vi "Control states_X-Y.vi"(7 "Command":T1(ring), 8 "error in (no error)":errorcluster, 10 "Reference in":refnum<vi>[](array[refnum])) -> (0 "error out":errorcluster)   [LabVIEW 2018]
doc: "This VI is used to enable & disable the controls"
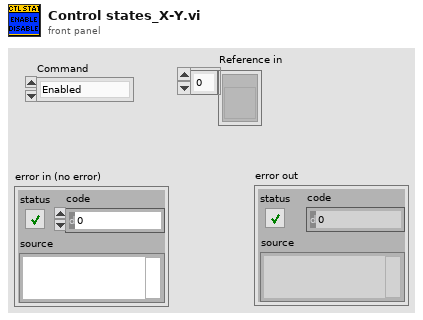
[diagram p1: front panel]
types:
  T1 = enum8{"Enabled", "Disabled", "Disabled and Grayed Out"}
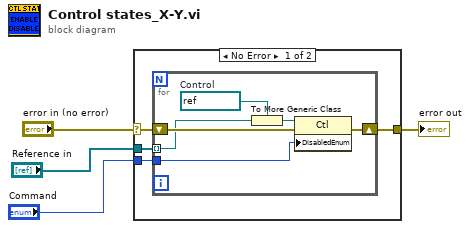
[diagram p0: block diagram]
diagram:
  n1 = case shown="No Error" "error in (no error)" {
    selector: "error in (no error)" -> [w8 w15]
    tunnel: [w7 w15] -> w3
    tunnel: "Reference in" -> [w6 _]
    tunnel: "Command" -> [w5 _]
    frame No Error {
      n2 = for {
        shift-right: [w13] -> w7
        shift-left: w8 -> [w14]
        tunnel: w6 -> [w11] mode=indexing
        tunnel: w5 -> [w9]
        w12 = refnum<vi> refnum  # Control
        n3 = To More Generic Class(target class=w12, reference=w11) -> (generic class reference=w10:refnum<vi>)
        n4 = property class="Ctl"(reference=w10, error in=w14, "DisabledEnum"=w9) -> (error out=w13:errorcluster)  [unwired: 1 out]
      }
    }
    frame Error {
    }
  }
  "error out" <- w3
